vi "CountdownTimer.vi"(0 "Stop Program":refnum<vi>, 2 "Countdown X":refnum<vi>) -> ()   [LabVIEW 2022 SP3]
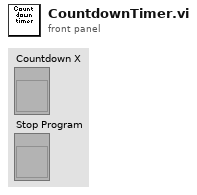
[diagram p1: front panel]
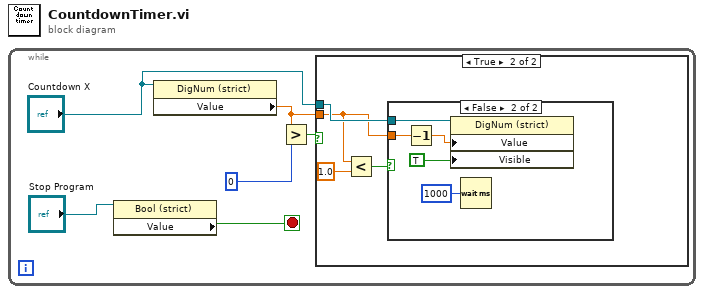
[diagram p0: block diagram]
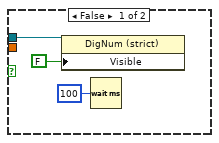
[diagram p2: hidden frame]
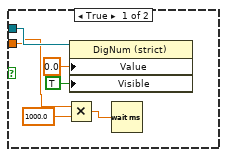
[diagram p3: hidden frame]
diagram:
  n1 = while {
    stop <- w1 stop-if-true
    n2 = property class="Bool (strict)"(reference="Stop Program") -> ("Value"=w1:bool)  [unwired: 1 in, 2 out]
    n3 = property class="DigNum (strict)"(reference="Countdown X") -> ("Value"=w4:dbl)  [unwired: 1 in, 2 out]
    n4 = Greater?(x=w4, y=0) -> (0:w5:bool)
    n5 = case shown="True" w5 {
      tunnel: "Countdown X" -> [w8 w13]
      tunnel: w4 -> [_ w11]
      frame False {
        n6 = property class="DigNum (strict)"(reference=w8, "Visible"=FALSE) -> ()  [unwired: 1 in, 2 out]
        n7 = Wait (ms)(milliseconds to wait=u32 100 ("millisecond multiple")) -> ()  [unwired: 1 out]
      }
      frame True {
        n8 = Less?(x=w11, y=1.0) -> (x < y?=w10:bool)
        n9 = case shown="False" w10 {
          tunnel: w13 -> [w18 w23]
          tunnel: w11 -> [w16 w22]
          frame True {
            n10 = Multiply(x=w16, y=1000.0) -> (x*y=w14:dbl)
            n11 = property class="DigNum (strict)"(reference=w18, "Value"=0.0, "Visible"=TRUE) -> ()  [unwired: 1 in, 2 out]
            n12 = Wait (ms)(milliseconds to wait=w14) -> ()  [unwired: 1 out]
          }
          frame False {
            n13 = Decrement(x=w22) -> (x-1=w21:dbl)
            n14 = property class="DigNum (strict)"(reference=w23, "Value"=w21, "Visible"=TRUE) -> ()  [unwired: 1 in, 2 out]
            n15 = Wait (ms)(milliseconds to wait=u32 1000 ("millisecond multiple")) -> ()  [unwired: 1 out]
          }
        }
      }
    }
  }
